vi "CAENHV Set Ch Param Bool.vi"(5 "ParValue":bool, 6 "ChList":u16[](array[numeric]), 7 "ChNum (1)":u16=1, 8 "error in (no error)":errorcluster, 9 "ParName":string, 10 "slot":u16, 11 "handle":i32) -> (0 "error out":errorcluster)   [LabVIEW 2018, in "CAENHVWrapper.lvlib"]
doc: "CAENHVLIB_API CAENHVRESULT CAENHV_SetChParam(int handle, ushort slot, \n const char *ParName, ushort ChNum, const ushort *ChList, void *ParValue);"
uses:
  <instrlib>/CAENHVWrapper/CAENHVWrapper.lvlib
  <instrlib>/CAENHVWrapper/VIs/CAENHVWrapper.dll
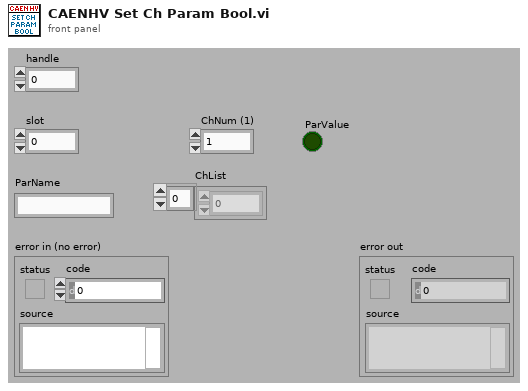
[diagram p1: front panel]
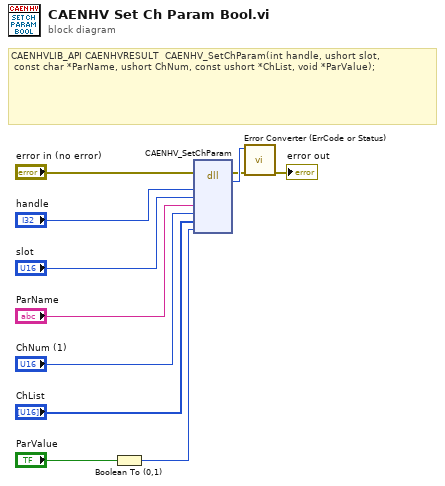
[diagram p0: block diagram]
diagram:
  # "CAENHVLIB_API CAENHVRESULT  CAENHV_SetChParam(int handle, ushort slot, \n const char *ParName, ushort ChNum, const ushort *ChList, void *ParValue);"
  n1 = Boolean To (0,1)(Boolean="ParValue") -> (0, 1=w2:i16)
  n2 = dll-call lib="C:/Program Files (x86)/National Instruments/LabVIEW 2018/instr.lib/CAENHVWrapper/VIs/CAENHVWrapper.*" fn="CAENHV_SetChParam"(error in="error in (no error)", "handle"="handle", "slot"="slot", "ParName"="ParName", "ChNum"="ChNum (1)", "ChList"="ChList", "ParValue"=w2) -> (error out=w4:errorcluster, "return type"=w5:i32)  [unwired: 8 in, 1 out]
  n3 = call <instrlib>:"Error Converter (ErrCode or Status).vi"("error in (no error)"=w4, "error code"=w5) -> ("error out"=→"error out":errorcluster)  [unwired: 9 in]
